vi "Master VI.vi"() -> ()   [LabVIEW 2010]
uses:
  <vilib>/Analysis/Matrix/Datatypes/RealMatrix.ctl
  Valve_Pump.ctl
  <vilib>/Analysis/Matrix/Comparison/Equal/Equal - RM,RM.vi
  <vilib>/Analysis/Matrix/NI_Matrix.lvlib
panel:
  in  "Density Profile":T1
  in  "Manual Override":bool
  in  "Drain Main Tank":bool
  in  "Open All":bool
  in  "Pump D":bool
  in  "V 37":bool
  in  "V 36":bool
  in  "V 35":bool
  in  "V 34":bool
  in  "V 32":bool
  in  "V 31":bool
  in  "V 28":bool
  in  "V 27":bool
  in  "V 26":bool
  in  "V 25":bool
  in  "V 24":bool
  in  "V 22":bool
  in  "V 21":bool
  in  "V 20":bool
  in  "V 18":bool
  in  "V 15":bool
  in  "V 14":bool
  in  "V 13":bool
  in  "V 12":bool
  in  "V 11":bool
  in  "V 10":bool
  in  "V 9":bool
  in  "V 8":bool
  in  "V 6":bool
  in  "V 5":bool
  in  "V 1":bool
  in  "Fill Main Tank":bool
  in  "V 23":bool
  in  "V 29":bool
  in  "V 30":bool
  in  "Pump A":bool
  out "Main tank":dbl(slide) scale=0.0..1.0
  out "Height of tank (m)":dbl
  out "Volume m^3*1000":i32
  in  "Reset":bool
  in  "Pump C":bool
  in  "Pump B":bool
  in  "V 19":bool
  in  "V 17":bool
  in  "V 16":bool
  in  "V 33":bool
  in  "V 3":bool
  in  "V 2":bool
  in  "V 4":bool
  in  "V 7":bool
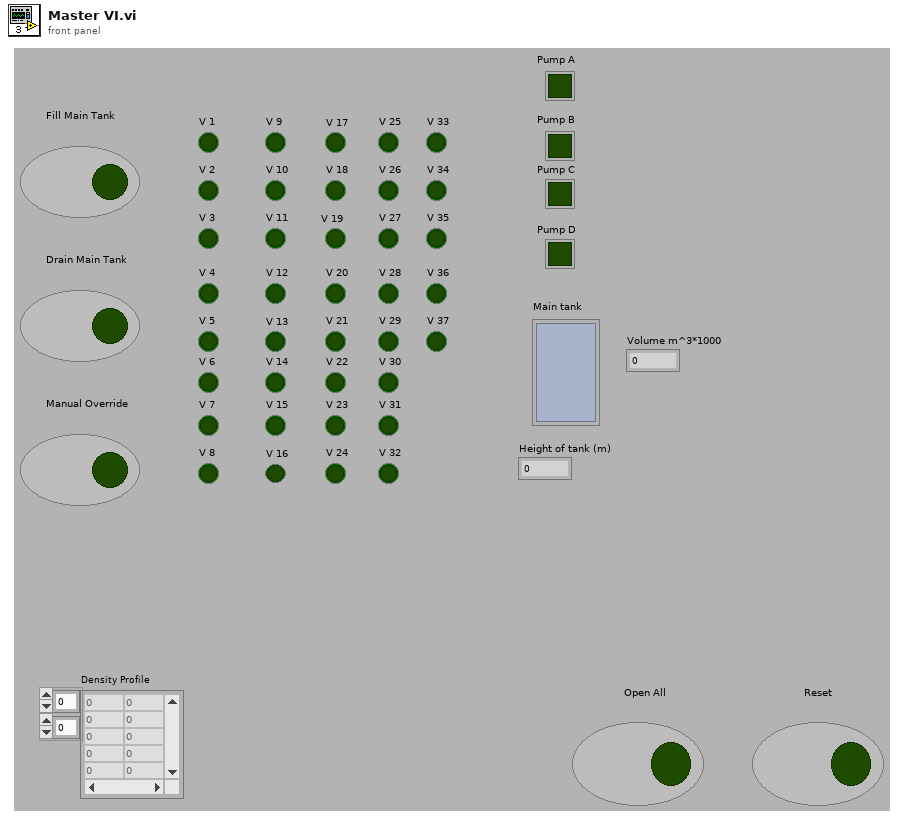
[diagram p1: front panel]
types:
  T1 = typedef "NI_Matrix.lvlib/RealMatrix.ctl" = dbl[][]
  T2 = typedef "Valve_Pump.ctl" = enum16{"V1", "V2", "V3", "V4", "V5", "V6", "V7", "V8", "V9", "V10", "V11", "V12", "V13", "V14", "V15", "V16", "V17", "V18", "V19", "V20", "V21", "V22", "V23", "V24", "V25", "V26", "V27", "V28", "V29", "V30", "V31", "V32", "V33", "V34", "V35", "V36", "V37", "Pump A", "Pump B", "Pump C", "Pump D"}
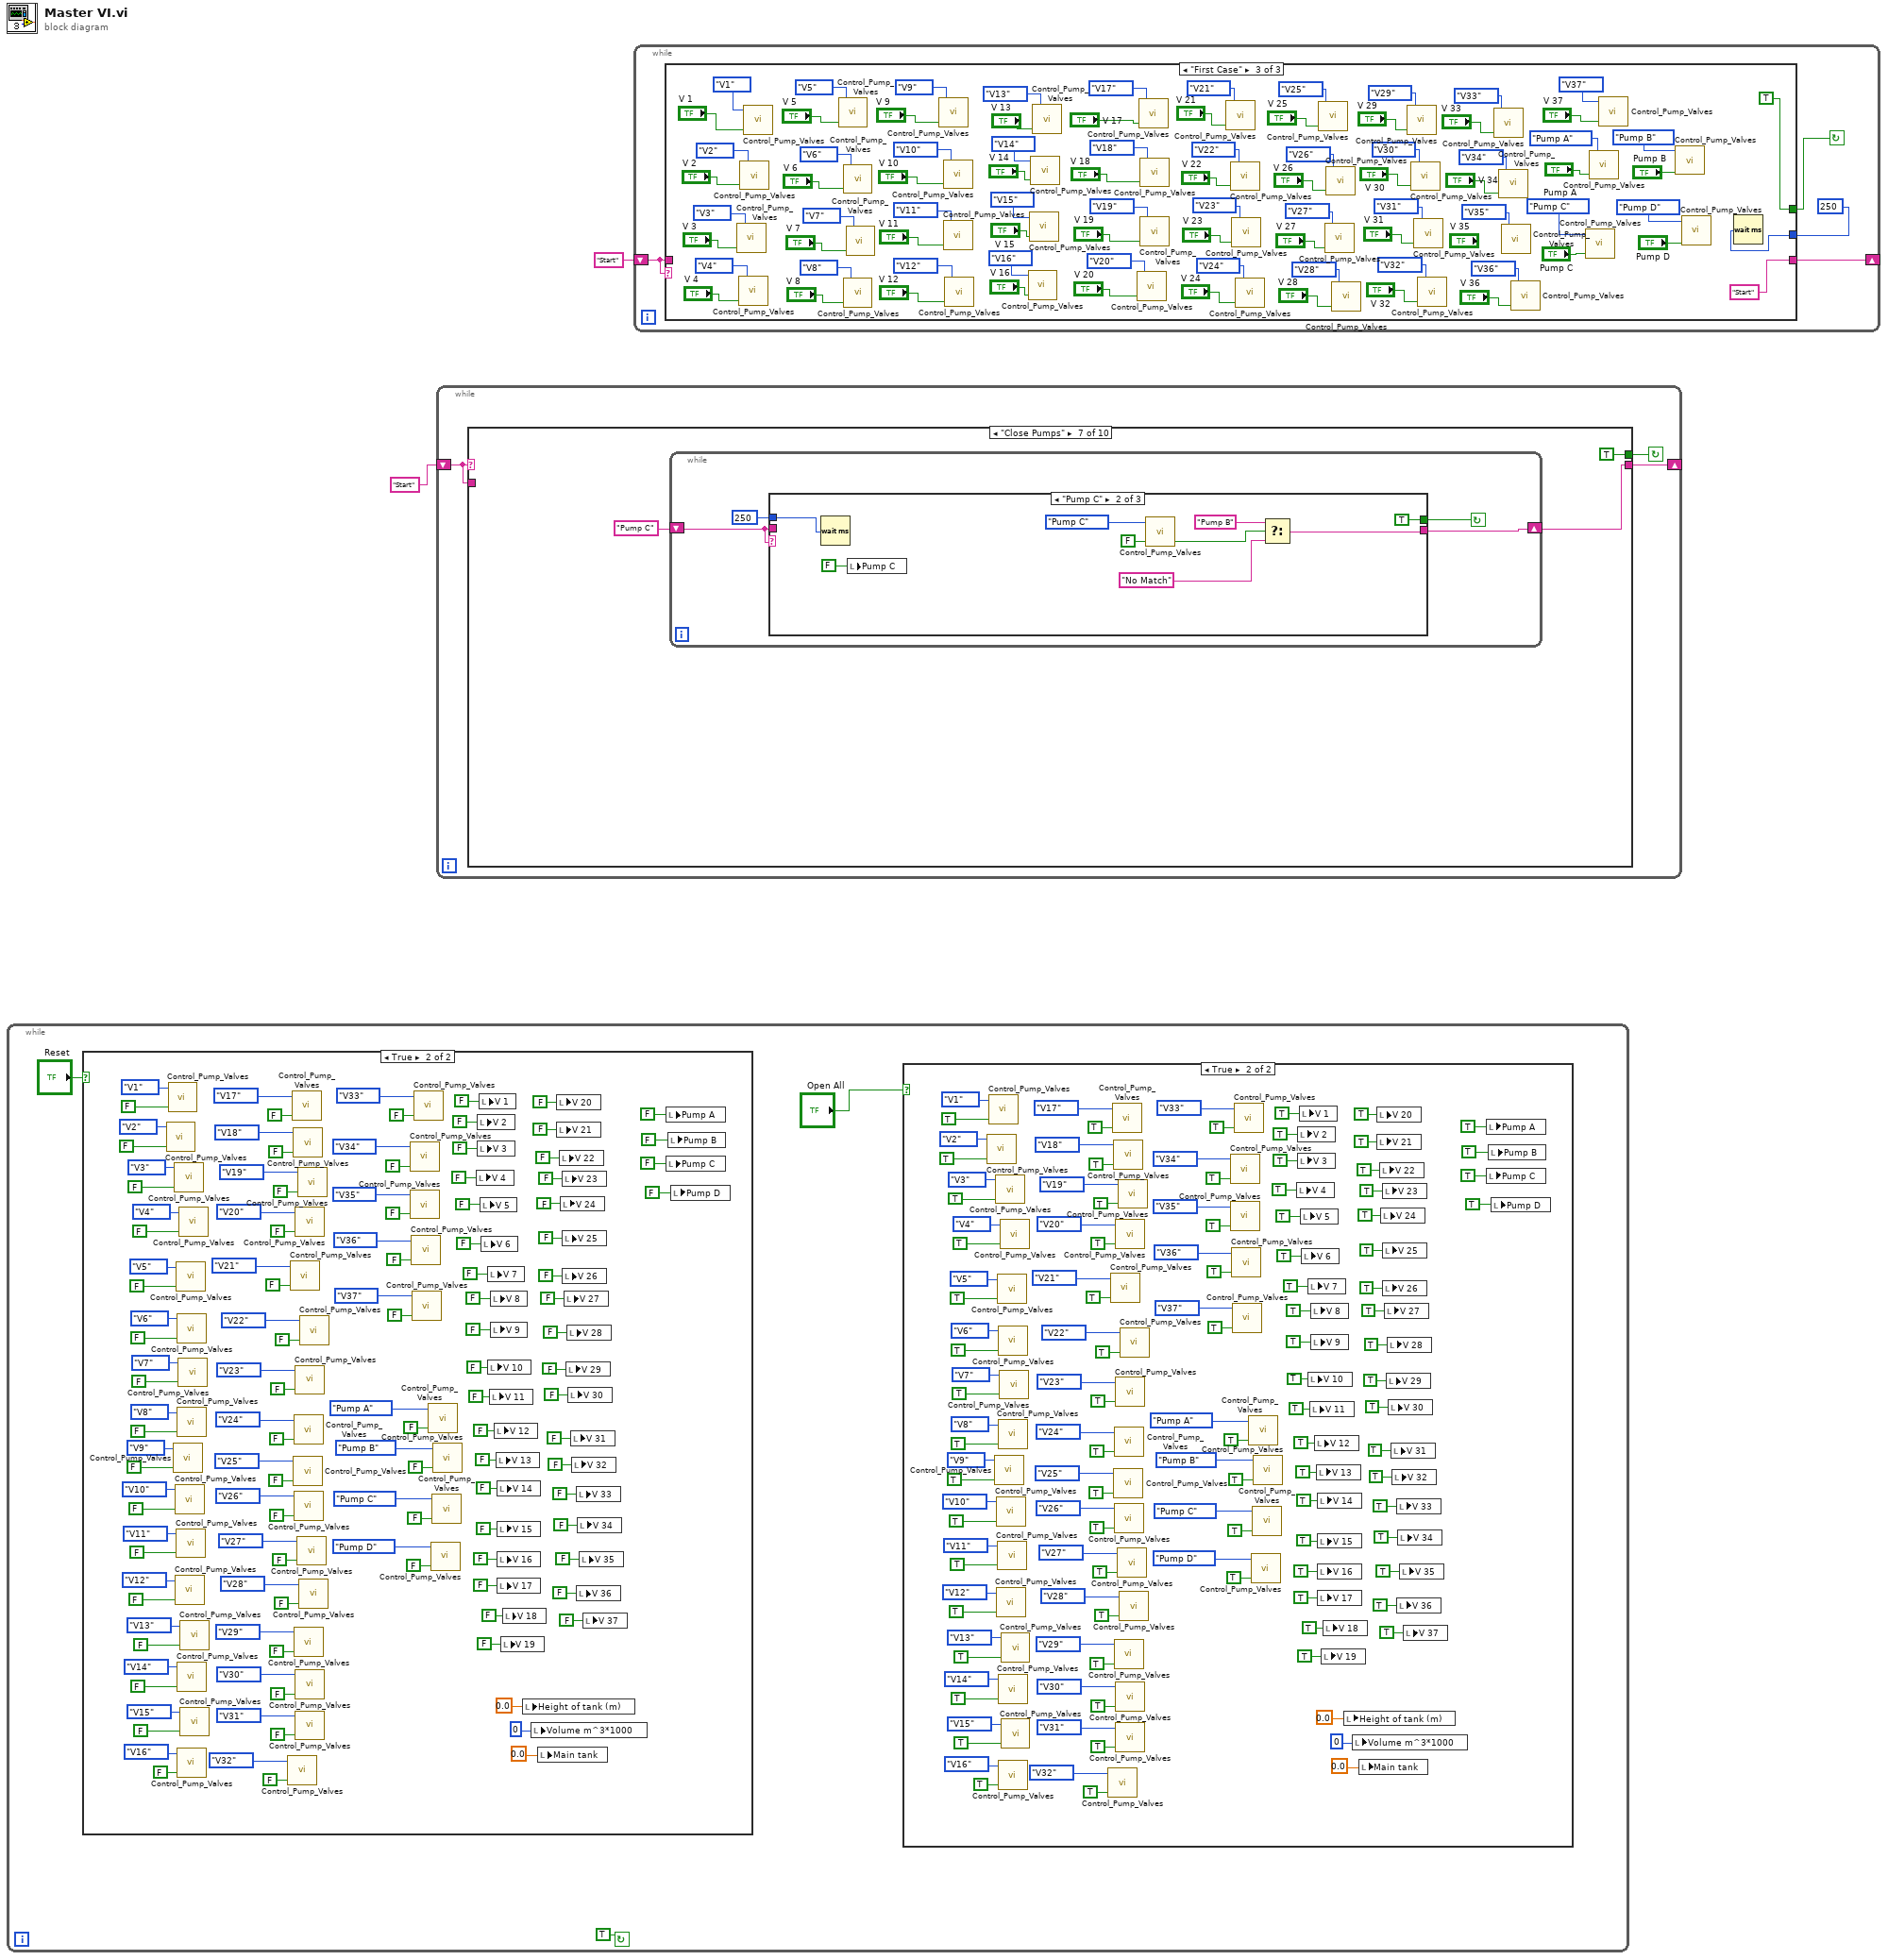
[diagram p0: block diagram]
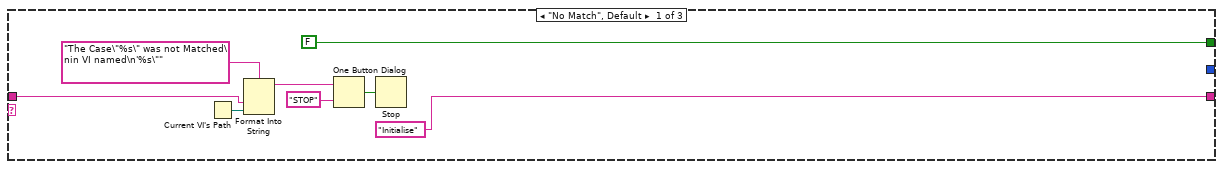
[diagram p2: hidden frame]
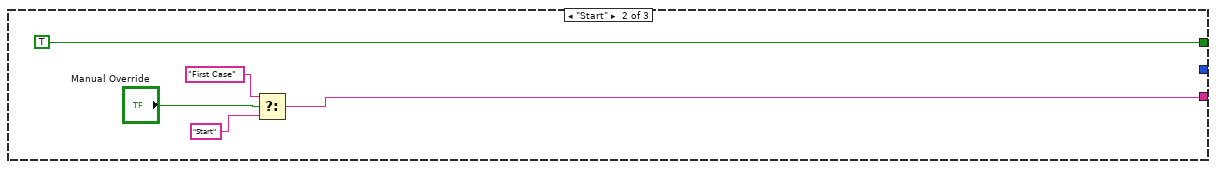
[diagram p3: hidden frame]
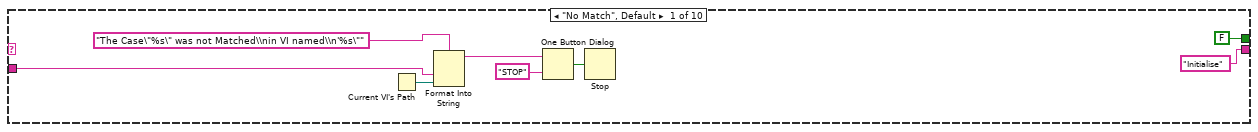
[diagram p6: hidden frame]
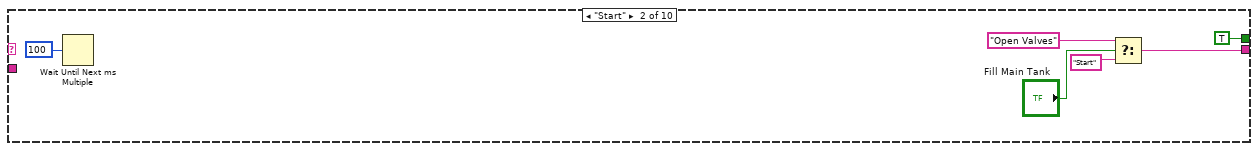
[diagram p7: hidden frame]
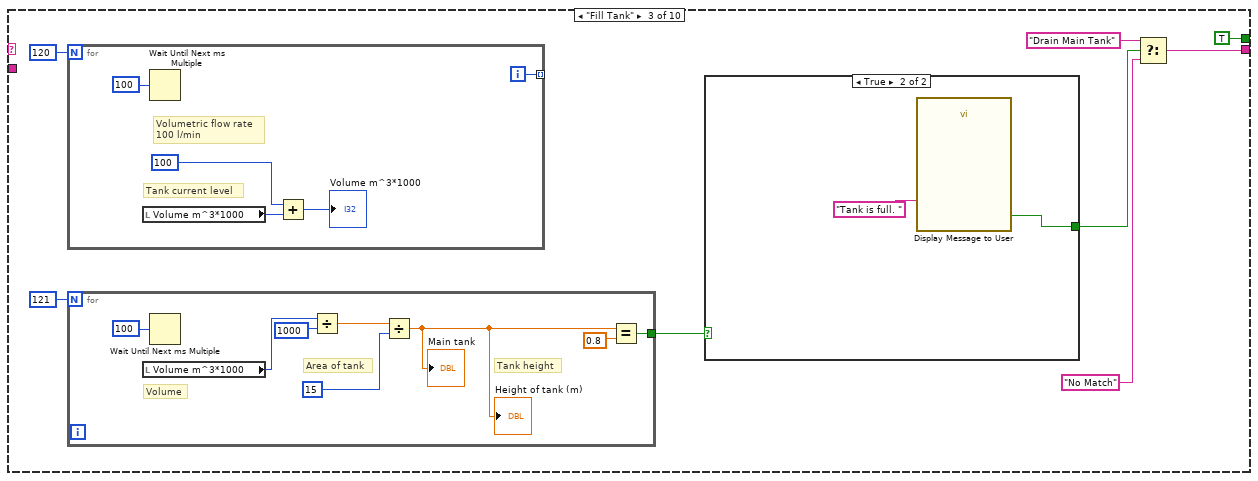
[diagram p8: hidden frame]
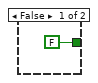
[diagram p9: hidden frame]
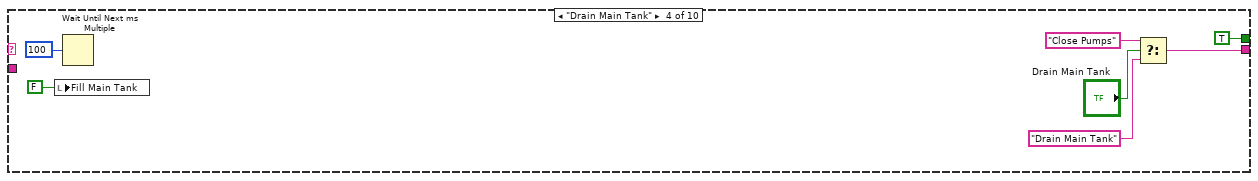
[diagram p10: hidden frame]
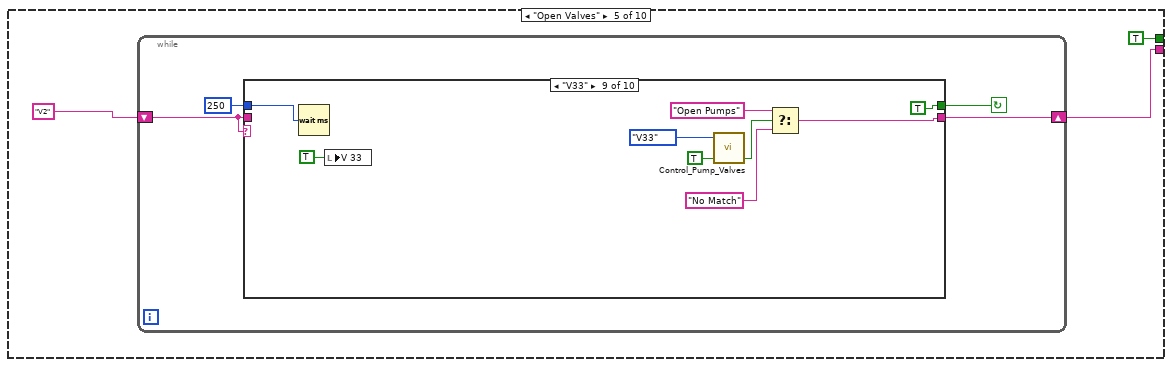
[diagram p11: hidden frame]
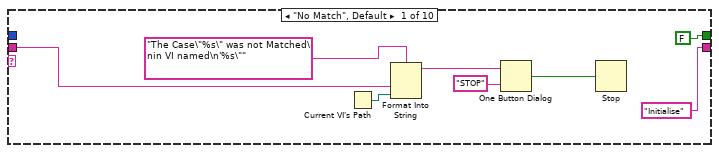
[diagram p12: hidden frame]
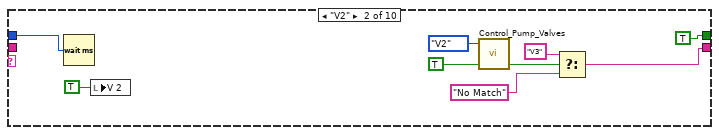
[diagram p13: hidden frame]
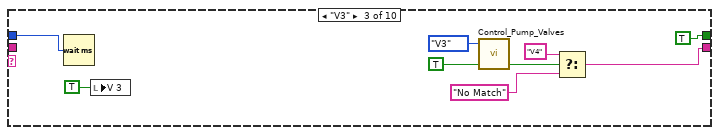
[diagram p14: hidden frame]
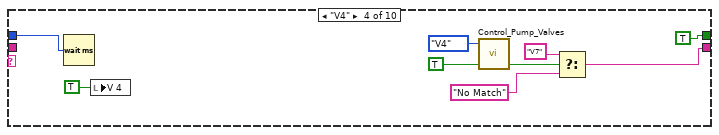
[diagram p15: hidden frame]
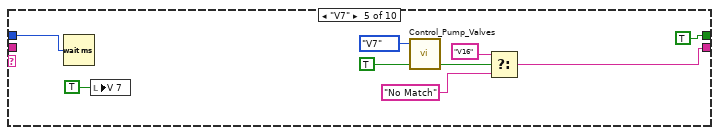
[diagram p16: hidden frame]
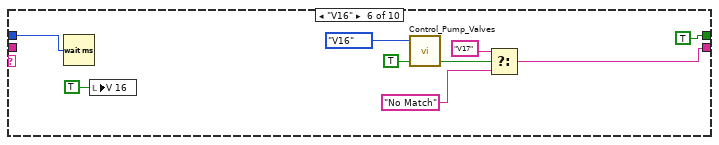
[diagram p17: hidden frame]
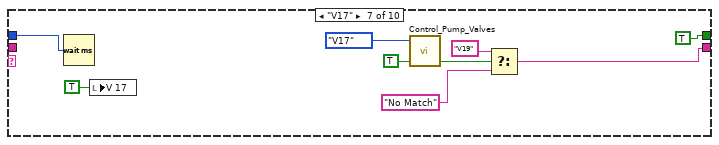
[diagram p18: hidden frame]
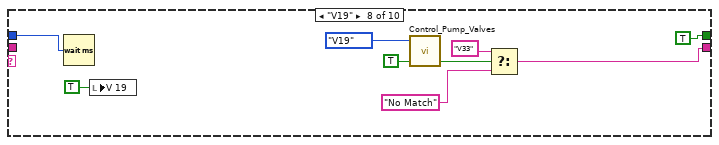
[diagram p19: hidden frame]
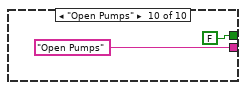
[diagram p20: hidden frame]
diagram:
  n1 = while {
    stop <- TRUE continue-if-true
    n2 = case shown="True" "Reset" {
      frame False {
      }
      frame True {
        n3 = call "Control_Pump_Valves.vi"("Set state:"=FALSE, "Device"=Valve_Pump."V2") -> ()  [unwired: 2 in, 2 out]
        n4 = call "Control_Pump_Valves.vi"("Set state:"=FALSE, "Device"=Valve_Pump."V1") -> ()  [unwired: 2 in, 2 out]
        n5 = call "Control_Pump_Valves.vi"("Set state:"=FALSE, "Device"=Valve_Pump."V9") -> ()  [unwired: 2 in, 2 out]
        n6 = call "Control_Pump_Valves.vi"("Set state:"=FALSE, "Device"=Valve_Pump."V3") -> ()  [unwired: 2 in, 2 out]
        n7 = call "Control_Pump_Valves.vi"("Set state:"=FALSE, "Device"=Valve_Pump."V10") -> ()  [unwired: 2 in, 2 out]
        n8 = call "Control_Pump_Valves.vi"("Set state:"=FALSE, "Device"=Valve_Pump."V12") -> ()  [unwired: 2 in, 2 out]
        n9 = call "Control_Pump_Valves.vi"("Set state:"=FALSE, "Device"=Valve_Pump."V5") -> ()  [unwired: 2 in, 2 out]
        n10 = call "Control_Pump_Valves.vi"("Set state:"=FALSE, "Device"=Valve_Pump."V11") -> ()  [unwired: 2 in, 2 out]
        n11 = call "Control_Pump_Valves.vi"("Set state:"=FALSE, "Device"=Valve_Pump."V6") -> ()  [unwired: 2 in, 2 out]
        n12 = call "Control_Pump_Valves.vi"("Set state:"=FALSE, "Device"=Valve_Pump."V8") -> ()  [unwired: 2 in, 2 out]
        n13 = call "Control_Pump_Valves.vi"("Set state:"=FALSE, "Device"=Valve_Pump."V14") -> ()  [unwired: 2 in, 2 out]
        n14 = call "Control_Pump_Valves.vi"("Set state:"=FALSE, "Device"=Valve_Pump."V16") -> ()  [unwired: 2 in, 2 out]
        n15 = call "Control_Pump_Valves.vi"("Set state:"=FALSE, "Device"=Valve_Pump."V7") -> ()  [unwired: 2 in, 2 out]
        n16 = call "Control_Pump_Valves.vi"("Set state:"=FALSE, "Device"=Valve_Pump."V4") -> ()  [unwired: 2 in, 2 out]
        n17 = call "Control_Pump_Valves.vi"("Set state:"=FALSE, "Device"=Valve_Pump."V13") -> ()  [unwired: 2 in, 2 out]
        n18 = call "Control_Pump_Valves.vi"("Set state:"=FALSE, "Device"=Valve_Pump."V15") -> ()  [unwired: 2 in, 2 out]
        n19 = call "Control_Pump_Valves.vi"("Set state:"=FALSE, "Device"=Valve_Pump."V32") -> ()  [unwired: 2 in, 2 out]
        n20 = call "Control_Pump_Valves.vi"("Set state:"=FALSE, "Device"=Valve_Pump."V21") -> ()  [unwired: 2 in, 2 out]
        n21 = call "Control_Pump_Valves.vi"("Set state:"=FALSE, "Device"=Valve_Pump."V17") -> ()  [unwired: 2 in, 2 out]
        n22 = call "Control_Pump_Valves.vi"("Set state:"=FALSE, "Device"=Valve_Pump."V18") -> ()  [unwired: 2 in, 2 out]
        n23 = call "Control_Pump_Valves.vi"("Set state:"=FALSE, "Device"=Valve_Pump."V25") -> ()  [unwired: 2 in, 2 out]
        n24 = call "Control_Pump_Valves.vi"("Set state:"=FALSE, "Device"=Valve_Pump."V24") -> ()  [unwired: 2 in, 2 out]
        n25 = call "Control_Pump_Valves.vi"("Set state:"=FALSE, "Device"=Valve_Pump."V26") -> ()  [unwired: 2 in, 2 out]
        n26 = call "Control_Pump_Valves.vi"("Set state:"=FALSE, "Device"=Valve_Pump."V29") -> ()  [unwired: 2 in, 2 out]
        n27 = call "Control_Pump_Valves.vi"("Set state:"=FALSE, "Device"=Valve_Pump."V20") -> ()  [unwired: 2 in, 2 out]
        n28 = call "Control_Pump_Valves.vi"("Set state:"=FALSE, "Device"=Valve_Pump."V23") -> ()  [unwired: 2 in, 2 out]
        n29 = call "Control_Pump_Valves.vi"("Set state:"=FALSE, "Device"=Valve_Pump."V30") -> ()  [unwired: 2 in, 2 out]
        n30 = call "Control_Pump_Valves.vi"("Set state:"=FALSE, "Device"=Valve_Pump."V31") -> ()  [unwired: 2 in, 2 out]
        n31 = call "Control_Pump_Valves.vi"("Set state:"=FALSE, "Device"=Valve_Pump."V27") -> ()  [unwired: 2 in, 2 out]
        n32 = call "Control_Pump_Valves.vi"("Set state:"=FALSE, "Device"=Valve_Pump."V19") -> ()  [unwired: 2 in, 2 out]
        n33 = call "Control_Pump_Valves.vi"("Set state:"=FALSE, "Device"=Valve_Pump."V28") -> ()  [unwired: 2 in, 2 out]
        n34 = call "Control_Pump_Valves.vi"("Set state:"=FALSE, "Device"=Valve_Pump."V22") -> ()  [unwired: 2 in, 2 out]
        n35 = call "Control_Pump_Valves.vi"("Set state:"=FALSE, "Device"=Valve_Pump."V34") -> ()  [unwired: 2 in, 2 out]
        n36 = call "Control_Pump_Valves.vi"("Set state:"=FALSE, "Device"=Valve_Pump."V35") -> ()  [unwired: 2 in, 2 out]
        n37 = call "Control_Pump_Valves.vi"("Set state:"=FALSE, "Device"=Valve_Pump."V36") -> ()  [unwired: 2 in, 2 out]
        n38 = call "Control_Pump_Valves.vi"("Set state:"=FALSE, "Device"=Valve_Pump."V37") -> ()  [unwired: 2 in, 2 out]
        n39 = call "Control_Pump_Valves.vi"("Set state:"=FALSE, "Device"=Valve_Pump."V33") -> ()  [unwired: 2 in, 2 out]
        n40 = call "Control_Pump_Valves.vi"("Set state:"=FALSE, "Device"=Valve_Pump."Pump A") -> ()  [unwired: 2 in, 2 out]
        n41 = call "Control_Pump_Valves.vi"("Set state:"=FALSE, "Device"=Valve_Pump."Pump D") -> ()  [unwired: 2 in, 2 out]
        n42 = call "Control_Pump_Valves.vi"("Set state:"=FALSE, "Device"=Valve_Pump."Pump C") -> ()  [unwired: 2 in, 2 out]
        n43 = call "Control_Pump_Valves.vi"("Set state:"=FALSE, "Device"=Valve_Pump."Pump B") -> ()  [unwired: 2 in, 2 out]
        n44 = local write "V 4"(FALSE ("V 4")) -> ()
        n45 = local write "V 2"(FALSE ("V 2")) -> ()
        n46 = local write "V 3"(FALSE ("V 3")) -> ()
        n47 = local write "V 1"(FALSE ("V 2")) -> ()
        n48 = local write "V 5"(FALSE ("V 3")) -> ()
        n49 = local write "V 6"(FALSE ("V 3")) -> ()
        n50 = local write "V 7"(FALSE ("V 7")) -> ()
        n51 = local write "V 10"(FALSE ("V 7")) -> ()
        n52 = local write "V 11"(FALSE ("V 7")) -> ()
        n53 = local write "V 8"(FALSE ("V 7")) -> ()
        n54 = local write "V 9"(FALSE ("V 7")) -> ()
        n55 = local write "V 12"(FALSE ("V 7")) -> ()
        n56 = local write "V 13"(FALSE ("V 7")) -> ()
        n57 = local write "V 14"(FALSE ("V 7")) -> ()
        n58 = local write "V 15"(FALSE ("V 7")) -> ()
        n59 = local write "V 16"(FALSE ("V 16")) -> ()
        n60 = local write "V 17"(FALSE ("V 17")) -> ()
        n61 = local write "V 19"(FALSE ("V 19")) -> ()
        n62 = local write "V 18"(FALSE ("V 7")) -> ()
        n63 = local write "Height of tank (m)"(0.0 ("Height of tank (m)")) -> ()
        n64 = local write "Volume m^3*1000"(0 ("Volume m^3*1000")) -> ()
        n65 = local write "Main tank"(0.0 ("Main tank")) -> ()
        n66 = local write "V 20"(FALSE ("V 19")) -> ()
        n67 = local write "V 21"(FALSE ("V 19")) -> ()
        n68 = local write "V 22"(FALSE ("V 19")) -> ()
        n69 = local write "V 24"(FALSE ("V 19")) -> ()
        n70 = local write "V 23"(FALSE ("V 19")) -> ()
        n71 = local write "V 25"(FALSE ("V 19")) -> ()
        n72 = local write "V 26"(FALSE ("V 19")) -> ()
        n73 = local write "V 27"(FALSE ("V 19")) -> ()
        n74 = local write "V 29"(FALSE ("V 19")) -> ()
        n75 = local write "V 28"(FALSE ("V 19")) -> ()
        n76 = local write "V 30"(FALSE ("V 19")) -> ()
        n77 = local write "V 31"(FALSE ("V 19")) -> ()
        n78 = local write "V 32"(FALSE ("V 33")) -> ()
        n79 = local write "V 33"(FALSE ("V 33")) -> ()
        n80 = local write "V 36"(FALSE ("V 19")) -> ()
        n81 = local write "V 34"(FALSE ("V 19")) -> ()
        n82 = local write "V 35"(FALSE ("V 19")) -> ()
        n83 = local write "V 37"(FALSE ("V 19")) -> ()
        n84 = local write "Pump A"(FALSE ("Pump B")) -> ()
        n85 = local write "Pump C"(FALSE ("Pump C")) -> ()
        n86 = local write "Pump B"(FALSE ("Pump B")) -> ()
        n87 = local write "Pump D"(FALSE ("Pump B")) -> ()
      }
    }
    n88 = case shown="True" "Open All" {
      frame False {
      }
      frame True {
        n89 = call "Control_Pump_Valves.vi"("Set state:"=TRUE, "Device"=Valve_Pump."V2") -> ()  [unwired: 2 in, 2 out]
        n90 = call "Control_Pump_Valves.vi"("Set state:"=TRUE, "Device"=Valve_Pump."V1") -> ()  [unwired: 2 in, 2 out]
        n91 = call "Control_Pump_Valves.vi"("Set state:"=TRUE, "Device"=Valve_Pump."V9") -> ()  [unwired: 2 in, 2 out]
        n92 = call "Control_Pump_Valves.vi"("Set state:"=TRUE, "Device"=Valve_Pump."V3") -> ()  [unwired: 2 in, 2 out]
        n93 = call "Control_Pump_Valves.vi"("Set state:"=TRUE, "Device"=Valve_Pump."V10") -> ()  [unwired: 2 in, 2 out]
        n94 = call "Control_Pump_Valves.vi"("Set state:"=TRUE, "Device"=Valve_Pump."V12") -> ()  [unwired: 2 in, 2 out]
        n95 = call "Control_Pump_Valves.vi"("Set state:"=TRUE, "Device"=Valve_Pump."V5") -> ()  [unwired: 2 in, 2 out]
        n96 = call "Control_Pump_Valves.vi"("Set state:"=TRUE, "Device"=Valve_Pump."V11") -> ()  [unwired: 2 in, 2 out]
        n97 = call "Control_Pump_Valves.vi"("Set state:"=TRUE, "Device"=Valve_Pump."V6") -> ()  [unwired: 2 in, 2 out]
        n98 = call "Control_Pump_Valves.vi"("Set state:"=TRUE, "Device"=Valve_Pump."V8") -> ()  [unwired: 2 in, 2 out]
        n99 = call "Control_Pump_Valves.vi"("Set state:"=TRUE, "Device"=Valve_Pump."V14") -> ()  [unwired: 2 in, 2 out]
        n100 = call "Control_Pump_Valves.vi"("Set state:"=TRUE, "Device"=Valve_Pump."V16") -> ()  [unwired: 2 in, 2 out]
        n101 = call "Control_Pump_Valves.vi"("Set state:"=TRUE, "Device"=Valve_Pump."V7") -> ()  [unwired: 2 in, 2 out]
        n102 = call "Control_Pump_Valves.vi"("Set state:"=TRUE, "Device"=Valve_Pump."V4") -> ()  [unwired: 2 in, 2 out]
        n103 = call "Control_Pump_Valves.vi"("Set state:"=TRUE, "Device"=Valve_Pump."V13") -> ()  [unwired: 2 in, 2 out]
        n104 = call "Control_Pump_Valves.vi"("Set state:"=TRUE, "Device"=Valve_Pump."V15") -> ()  [unwired: 2 in, 2 out]
        n105 = call "Control_Pump_Valves.vi"("Set state:"=TRUE, "Device"=Valve_Pump."V32") -> ()  [unwired: 2 in, 2 out]
        n106 = call "Control_Pump_Valves.vi"("Set state:"=TRUE, "Device"=Valve_Pump."V21") -> ()  [unwired: 2 in, 2 out]
        n107 = call "Control_Pump_Valves.vi"("Set state:"=TRUE, "Device"=Valve_Pump."V17") -> ()  [unwired: 2 in, 2 out]
        n108 = call "Control_Pump_Valves.vi"("Set state:"=TRUE, "Device"=Valve_Pump."V18") -> ()  [unwired: 2 in, 2 out]
        n109 = call "Control_Pump_Valves.vi"("Set state:"=TRUE, "Device"=Valve_Pump."V25") -> ()  [unwired: 2 in, 2 out]
        n110 = call "Control_Pump_Valves.vi"("Set state:"=TRUE, "Device"=Valve_Pump."V24") -> ()  [unwired: 2 in, 2 out]
        n111 = call "Control_Pump_Valves.vi"("Set state:"=TRUE, "Device"=Valve_Pump."V26") -> ()  [unwired: 2 in, 2 out]
        n112 = call "Control_Pump_Valves.vi"("Set state:"=TRUE, "Device"=Valve_Pump."V29") -> ()  [unwired: 2 in, 2 out]
        n113 = call "Control_Pump_Valves.vi"("Set state:"=TRUE, "Device"=Valve_Pump."V20") -> ()  [unwired: 2 in, 2 out]
        n114 = call "Control_Pump_Valves.vi"("Set state:"=TRUE, "Device"=Valve_Pump."V23") -> ()  [unwired: 2 in, 2 out]
        n115 = call "Control_Pump_Valves.vi"("Set state:"=TRUE, "Device"=Valve_Pump."V30") -> ()  [unwired: 2 in, 2 out]
        n116 = call "Control_Pump_Valves.vi"("Set state:"=TRUE, "Device"=Valve_Pump."V31") -> ()  [unwired: 2 in, 2 out]
        n117 = call "Control_Pump_Valves.vi"("Set state:"=TRUE, "Device"=Valve_Pump."V27") -> ()  [unwired: 2 in, 2 out]
        n118 = call "Control_Pump_Valves.vi"("Set state:"=TRUE, "Device"=Valve_Pump."V19") -> ()  [unwired: 2 in, 2 out]
        n119 = call "Control_Pump_Valves.vi"("Set state:"=TRUE, "Device"=Valve_Pump."V28") -> ()  [unwired: 2 in, 2 out]
        n120 = call "Control_Pump_Valves.vi"("Set state:"=TRUE, "Device"=Valve_Pump."V22") -> ()  [unwired: 2 in, 2 out]
        n121 = call "Control_Pump_Valves.vi"("Set state:"=TRUE, "Device"=Valve_Pump."V34") -> ()  [unwired: 2 in, 2 out]
        n122 = call "Control_Pump_Valves.vi"("Set state:"=TRUE, "Device"=Valve_Pump."V35") -> ()  [unwired: 2 in, 2 out]
        n123 = call "Control_Pump_Valves.vi"("Set state:"=TRUE, "Device"=Valve_Pump."V36") -> ()  [unwired: 2 in, 2 out]
        n124 = call "Control_Pump_Valves.vi"("Set state:"=TRUE, "Device"=Valve_Pump."V37") -> ()  [unwired: 2 in, 2 out]
        n125 = call "Control_Pump_Valves.vi"("Set state:"=TRUE, "Device"=Valve_Pump."V33") -> ()  [unwired: 2 in, 2 out]
        n126 = call "Control_Pump_Valves.vi"("Set state:"=TRUE, "Device"=Valve_Pump."Pump A") -> ()  [unwired: 2 in, 2 out]
        n127 = call "Control_Pump_Valves.vi"("Set state:"=TRUE, "Device"=Valve_Pump."Pump D") -> ()  [unwired: 2 in, 2 out]
        n128 = call "Control_Pump_Valves.vi"("Set state:"=TRUE, "Device"=Valve_Pump."Pump C") -> ()  [unwired: 2 in, 2 out]
        n129 = call "Control_Pump_Valves.vi"("Set state:"=TRUE, "Device"=Valve_Pump."Pump B") -> ()  [unwired: 2 in, 2 out]
        n130 = local write "V 4"(TRUE ("V 4")) -> ()
        n131 = local write "V 2"(TRUE ("V 2")) -> ()
        n132 = local write "V 3"(TRUE ("V 3")) -> ()
        n133 = local write "V 1"(TRUE ("V 2")) -> ()
        n134 = local write "V 5"(TRUE ("V 3")) -> ()
        n135 = local write "V 6"(TRUE ("V 3")) -> ()
        n136 = local write "V 7"(TRUE ("V 7")) -> ()
        n137 = local write "V 10"(TRUE ("V 7")) -> ()
        n138 = local write "V 11"(TRUE ("V 7")) -> ()
        n139 = local write "V 8"(TRUE ("V 7")) -> ()
        n140 = local write "V 9"(TRUE ("V 7")) -> ()
        n141 = local write "V 12"(TRUE ("V 7")) -> ()
        n142 = local write "V 13"(TRUE ("V 7")) -> ()
        n143 = local write "V 14"(TRUE ("V 7")) -> ()
        n144 = local write "V 15"(TRUE ("V 7")) -> ()
        n145 = local write "V 16"(TRUE ("V 16")) -> ()
        n146 = local write "V 17"(TRUE ("V 17")) -> ()
        n147 = local write "V 19"(TRUE ("V 19")) -> ()
        n148 = local write "V 18"(TRUE ("V 7")) -> ()
        n149 = local write "Height of tank (m)"(0.0 ("Height of tank (m)")) -> ()
        n150 = local write "Volume m^3*1000"(0 ("Volume m^3*1000")) -> ()
        n151 = local write "Main tank"(0.0 ("Main tank")) -> ()
        n152 = local write "V 20"(TRUE ("V 19")) -> ()
        n153 = local write "V 21"(TRUE ("V 19")) -> ()
        n154 = local write "V 22"(TRUE ("V 19")) -> ()
        n155 = local write "V 24"(TRUE ("V 19")) -> ()
        n156 = local write "V 23"(TRUE ("V 19")) -> ()
        n157 = local write "V 25"(TRUE ("V 19")) -> ()
        n158 = local write "V 26"(TRUE ("V 19")) -> ()
        n159 = local write "V 27"(TRUE ("V 19")) -> ()
        n160 = local write "V 29"(TRUE ("V 19")) -> ()
        n161 = local write "V 28"(TRUE ("V 19")) -> ()
        n162 = local write "V 30"(TRUE ("V 19")) -> ()
        n163 = local write "V 31"(TRUE ("V 19")) -> ()
        n164 = local write "V 32"(TRUE ("V 33")) -> ()
        n165 = local write "V 33"(TRUE ("V 33")) -> ()
        n166 = local write "V 36"(TRUE ("V 19")) -> ()
        n167 = local write "V 34"(TRUE ("V 19")) -> ()
        n168 = local write "V 35"(TRUE ("V 19")) -> ()
        n169 = local write "V 37"(TRUE ("V 19")) -> ()
        n170 = local write "Pump A"(TRUE ("Pump B")) -> ()
        n171 = local write "Pump C"(TRUE ("Pump C")) -> ()
        n172 = local write "Pump B"(TRUE ("Pump B")) -> ()
        n173 = local write "Pump D"(TRUE ("Pump B")) -> ()
      }
    }
  }
  n174 = while {
    shift-left: "Start" -> [w258]
    shift-right: [w259] -> _
    stop <- w260 continue-if-true
    n175 = case shown="\"Close Pumps\"" w258 {
      tunnel: [FALSE TRUE TRUE TRUE TRUE TRUE TRUE TRUE TRUE TRUE] -> w260
      tunnel: ["Initialise" w271 w275 w301 w306 w395 w436 w469 w583 w607] -> w259
      tunnel: w258 -> [w263 _ _ _ _ _ _ _ _ _]
      frame "No Match", Default {
        n176 = Current VI's Path() -> (path=w262:path)
        n177 = Format Into String(format string="The Case\"%s\" was not Matched\\nin VI named\\n'%s\"" ("Format String"), w263, w262) -> (resulting string=w266:string)  [unwired: 2 in, 1 out]
        n178 = One Button Dialog(message=w266, button name ("OK")="STOP") -> (true=w264:bool)
        n179 = Stop(stop? (T)=w264) -> ()
      }
      frame "Start" {
        n180 = Wait Until Next ms Multiple(millisecond multiple=u32 100) -> ()  [unwired: 1 out]
        n181 = Select(t="Open Valves", s="Fill Main Tank", f="Start") -> (s? t:f=w271:string)
      }
      frame "Fill Tank" {
        n182 = for {
          N: 120 -> [_]
          tunnel: [w294] -> _ mode=indexing
          i -> [w294]
          # "Tank current level"
          # "Volumetric flow rate\n100 l/min"
          n183 = local read "Volume m^3*1000"() -> (w297:i32)
          n184 = Wait Until Next ms Multiple(millisecond multiple=u32 100) -> ()  [unwired: 1 out]
          n185 = Add(x=100, y=w297) -> (x+y=→"Volume m^3*1000":i32)
        }
        n186 = for {
          N: 121 -> [_]
          tunnel: [w283] -> w281
          # "Volume"
          # "Tank height"
          # "Area of tank"
          n187 = local read "Volume m^3*1000"() -> (w289:i32)
          n188 = Wait Until Next ms Multiple(millisecond multiple=u32 100 ("milliseconds to wait")) -> ()  [unwired: 1 out]
          n189 = Divide(x=w289, y=1000) -> (x/y=w287:dbl)
          n190 = Divide(x=w287, y=15) -> (x/y=w284:dbl)
          "Main tank" <- w284
          "Height of tank (m)" <- w284
          n191 = Equal?(x=w284, y=0.8) -> (x = y?=w283:bool)
        }
        n192 = case shown="True" w281 {
          tunnel: [FALSE ("OK") w292] -> w278
          frame False {
          }
          frame True {
            n193 = call "Display Message to User"("Message"="Tank is full. ") -> ("OK"=w292:bool)  [unwired: 9 in, 1 out]
          }
        }
        n194 = Select(t="Drain Main Tank" ("Message"), s=w278, f="No Match" ("Message")) -> (s? t:f=w275:string)
      }
      frame "Drain Main Tank" {
        n195 = local write "Fill Main Tank"(FALSE ("Fill Main Tank")) -> ()
        n196 = Wait Until Next ms Multiple(millisecond multiple=u32 100) -> ()  [unwired: 1 out]
        n197 = Select(t="Close Pumps", s="Drain Main Tank", f="Drain Main Tank") -> (s? t:f=w301:string)
      }
      frame "Open Valves" {
        n198 = while {
          shift-left: "V2" -> [w310]
          shift-right: [w311] -> w306
          stop <- w312 continue-if-true
          n199 = case shown="\"V33\"" w310 {
            tunnel: [FALSE TRUE TRUE TRUE TRUE TRUE TRUE TRUE TRUE FALSE] -> w312
            tunnel: ["Initialise" w323 w332 w341 w350 w359 w368 w377 w386 "Open Pumps" ("Message")] -> w311
            tunnel: w310 -> [w315 _ _ _ _ _ _ _ _ _]
            tunnel: u32 250 ("milliseconds to wait") -> [_ w327 w335 w344 w353 w362 w371 w380 w389 _]
            frame "No Match", Default {
              n200 = Current VI's Path() -> (path=w314:path)
              n201 = Format Into String(format string="The Case\"%s\" was not Matched\nin VI named\n'%s\"" ("Format String"), w315, w314) -> (resulting string=w318:string)  [unwired: 2 in, 1 out]
              n202 = One Button Dialog(message=w318, button name ("OK")="STOP") -> (true=w316:bool)
              n203 = Stop(stop? (T)=w316) -> ()
            }
            frame "V2" {
              n204 = Wait (ms)(milliseconds to wait=w327) -> ()  [unwired: 1 out]
              n205 = local write "V 2"(TRUE ("V 2")) -> ()
              n206 = call "Control_Pump_Valves.vi"("Set state:"=TRUE, "Device"=Valve_Pump."V2") -> ("Good Reply"=w322:bool)  [unwired: 2 in, 1 out]
              n207 = Select(t="V3", s=w322, f="No Match" ("Message")) -> (s? t:f=w323:string)
            }
            frame "V3" {
              n208 = Wait (ms)(milliseconds to wait=w335) -> ()  [unwired: 1 out]
              n209 = local write "V 3"(TRUE ("V 3")) -> ()
              n210 = call "Control_Pump_Valves.vi"("Set state:"=TRUE, "Device"=Valve_Pump."V3") -> ("Good Reply"=w331:bool)  [unwired: 2 in, 1 out]
              n211 = Select(t="V4", s=w331, f="No Match" ("Message")) -> (s? t:f=w332:string)
            }
            frame "V4" {
              n212 = Wait (ms)(milliseconds to wait=w344) -> ()  [unwired: 1 out]
              n213 = local write "V 4"(TRUE ("V 4")) -> ()
              n214 = call "Control_Pump_Valves.vi"("Set state:"=TRUE, "Device"=Valve_Pump."V4") -> ("Good Reply"=w340:bool)  [unwired: 2 in, 1 out]
              n215 = Select(t="V7", s=w340, f="No Match" ("Message")) -> (s? t:f=w341:string)
            }
            frame "V7" {
              n216 = Wait (ms)(milliseconds to wait=w353) -> ()  [unwired: 1 out]
              n217 = local write "V 7"(TRUE ("V 7")) -> ()
              n218 = call "Control_Pump_Valves.vi"("Set state:"=TRUE, "Device"=Valve_Pump."V7") -> ("Good Reply"=w349:bool)  [unwired: 2 in, 1 out]
              n219 = Select(t="V16", s=w349, f="No Match" ("Message")) -> (s? t:f=w350:string)
            }
            frame "V16" {
              n220 = Wait (ms)(milliseconds to wait=w362) -> ()  [unwired: 1 out]
              n221 = local write "V 16"(TRUE ("V 3")) -> ()
              n222 = call "Control_Pump_Valves.vi"("Set state:"=TRUE, "Device"=Valve_Pump."V16") -> ("Good Reply"=w358:bool)  [unwired: 2 in, 1 out]
              n223 = Select(t="V17", s=w358, f="No Match" ("Message")) -> (s? t:f=w359:string)
            }
            frame "V17" {
              n224 = Wait (ms)(milliseconds to wait=w371) -> ()  [unwired: 1 out]
              n225 = local write "V 17"(TRUE ("V 3")) -> ()
              n226 = call "Control_Pump_Valves.vi"("Set state:"=TRUE, "Device"=Valve_Pump."V17") -> ("Good Reply"=w367:bool)  [unwired: 2 in, 1 out]
              n227 = Select(t="V19", s=w367, f="No Match" ("Message")) -> (s? t:f=w368:string)
            }
            frame "V19" {
              n228 = Wait (ms)(milliseconds to wait=w380) -> ()  [unwired: 1 out]
              n229 = local write "V 19"(TRUE ("V 3")) -> ()
              n230 = call "Control_Pump_Valves.vi"("Set state:"=TRUE, "Device"=Valve_Pump."V19") -> ("Good Reply"=w376:bool)  [unwired: 2 in, 1 out]
              n231 = Select(t="V33", s=w376, f="No Match" ("Message")) -> (s? t:f=w377:string)
            }
            frame "V33" {
              n232 = Wait (ms)(milliseconds to wait=w389) -> ()  [unwired: 1 out]
              n233 = local write "V 33"(TRUE ("V 3")) -> ()
              n234 = call "Control_Pump_Valves.vi"("Set state:"=TRUE, "Device"=Valve_Pump."V33") -> ("Good Reply"=w385:bool)  [unwired: 2 in, 1 out]
              n235 = Select(t="Open Pumps", s=w385, f="No Match" ("Message")) -> (s? t:f=w386:string)
            }
            frame "Open Pumps" {
            }
          }
        }
      }
      frame "Open Pumps" {
        n236 = while {
          shift-left: "Pump B" -> [w399]
          shift-right: [w400] -> w395
          stop <- w401 continue-if-true
          n237 = case shown="\"Pump C\"" w399 {
            tunnel: [FALSE TRUE TRUE FALSE] -> w401
            tunnel: ["Initialise" w412 w421 w431] -> w400
            tunnel: w399 -> [w404 _ _ _]
            tunnel: u32 250 ("milliseconds to wait") -> [_ w416 w424 w434]
            frame "No Match", Default {
              n238 = Current VI's Path() -> (path=w403:path)
              n239 = Format Into String(format string="The Case\"%s\" was not Matched\nin VI named\n'%s\"" ("Format String"), w404, w403) -> (resulting string=w407:string)  [unwired: 2 in, 1 out]
              n240 = One Button Dialog(message=w407, button name ("OK")="STOP") -> (true=w405:bool)
              n241 = Stop(stop? (T)=w405) -> ()
            }
            frame "Pump B" {
              n242 = Wait (ms)(milliseconds to wait=w416) -> ()  [unwired: 1 out]
              n243 = local write "Pump B"(TRUE ("Pump B")) -> ()
              n244 = call "Control_Pump_Valves.vi"("Set state:"=TRUE, "Device"=Valve_Pump."Pump B") -> ("Good Reply"=w411:bool)  [unwired: 2 in, 1 out]
              n245 = Select(t="Pump C", s=w411, f="No Match" ("Message")) -> (s? t:f=w412:string)
            }
            frame "Pump C" {
              n246 = Wait (ms)(milliseconds to wait=w424) -> ()  [unwired: 1 out]
              n247 = local write "Pump C"(TRUE ("Pump B")) -> ()
              n248 = call "Control_Pump_Valves.vi"("Set state:"=TRUE, "Device"=Valve_Pump."Pump C") -> ("Good Reply"=w420:bool)  [unwired: 2 in, 1 out]
              n249 = Select(t="Density Profile", s=w420, f="No Match" ("Message")) -> (s? t:f=w421:string)
            }
            frame "Density Profile" {
              n250 = Wait (ms)(milliseconds to wait=w434) -> ()  [unwired: 1 out]
              n251 = call-poly <vilib>:"Equal.vi"("Real Matrix B"=T1 [[1200.0, 0.0], [1150.0, 0.2], [1100.0, 0.4], [1050.0, 0.6], [1000.0, 0.8]] ("Density Profile 2"), "Real Matrix A"="Density Profile") -> ("A = B?"=w428:bool)
              n252 = Select(t="Fill Tank", s=w428, f="No Match" ("Message")) -> (s? t:f=w431:string)
            }
          }
        }
      }
      frame "Close Pumps" {
        n253 = while {
          shift-left: "Pump C" -> [w440]
          shift-right: [w441] -> w436
          stop <- w442 continue-if-true
          n254 = case shown="\"Pump C\"" w440 {
            tunnel: [FALSE TRUE FALSE] -> w442
            tunnel: ["Initialise" w453 w462] -> w441
            tunnel: w440 -> [w445 _ _]
            tunnel: u32 250 ("milliseconds to wait") -> [_ w456 w466]
            frame "No Match", Default {
              n255 = Current VI's Path() -> (path=w444:path)
              n256 = Format Into String(format string="The Case\"%s\" was not Matched\nin VI named\n'%s\"" ("Format String"), w445, w444) -> (resulting string=w448:string)  [unwired: 2 in, 1 out]
              n257 = One Button Dialog(message=w448, button name ("OK")="STOP") -> (true=w446:bool)
              n258 = Stop(stop? (T)=w446) -> ()
            }
            frame "Pump C" {
              n259 = Wait (ms)(milliseconds to wait=w456) -> ()  [unwired: 1 out]
              n260 = local write "Pump C"(FALSE ("Pump B")) -> ()
              n261 = call "Control_Pump_Valves.vi"("Set state:"=FALSE, "Device"=Valve_Pump."Pump C") -> ("Good Reply"=w452:bool)  [unwired: 2 in, 1 out]
              n262 = Select(t="Pump B", s=w452, f="No Match" ("Message")) -> (s? t:f=w453:string)
            }
            frame "Pump B" {
              n263 = Wait (ms)(milliseconds to wait=w466) -> ()  [unwired: 1 out]
              n264 = local write "Pump B"(FALSE ("Pump B")) -> ()
              n265 = call "Control_Pump_Valves.vi"("Set state:"=FALSE, "Device"=Valve_Pump."Pump B") -> ("Good Reply"=w461:bool)  [unwired: 2 in, 1 out]
              n266 = Select(t="Close Valves", s=w461, f="No Match" ("Message")) -> (s? t:f=w462:string)
            }
          }
        }
      }
      frame "Close Valves" {
        n267 = while {
          shift-left: "V2" -> [w473]
          shift-right: [w474] -> w469
          stop <- w475 continue-if-true
          n268 = case shown="\"Pump A\"" w473 {
            tunnel: [FALSE TRUE TRUE TRUE TRUE TRUE TRUE TRUE TRUE TRUE TRUE FALSE] -> w475
            tunnel: ["Initialise" w486 w495 w504 w513 w522 w531 w540 w549 w558 w567 w576] -> w474
            tunnel: w473 -> [w478 _ _ _ _ _ _ _ _ _ _ _]
            tunnel: u32 250 ("milliseconds to wait") -> [_ w489 w499 w508 w517 w526 w535 w544 w553 w562 w571 w580]
            frame "No Match", Default {
              n269 = Current VI's Path() -> (path=w477:path)
              n270 = Format Into String(format string="The Case\"%s\" was not Matched\nin VI named\n'%s\"" ("Format String"), w478, w477) -> (resulting string=w481:string)  [unwired: 2 in, 1 out]
              n271 = One Button Dialog(message=w481, button name ("OK")="STOP") -> (true=w479:bool)
              n272 = Stop(stop? (T)=w479) -> ()
            }
            frame "V2" {
              n273 = Wait (ms)(milliseconds to wait=w489) -> ()  [unwired: 1 out]
              n274 = local write "V 2"(FALSE ("V 4")) -> ()
              n275 = call "Control_Pump_Valves.vi"("Set state:"=FALSE, "Device"=Valve_Pump."V2") -> ("Good Reply"=w485:bool)  [unwired: 2 in, 1 out]
              n276 = Select(t="V3", s=w485, f="No Match" ("Message")) -> (s? t:f=w486:string)
            }
            frame "V3" {
              n277 = Wait (ms)(milliseconds to wait=w499) -> ()  [unwired: 1 out]
              n278 = local write "V 3"(FALSE ("V 3")) -> ()
              n279 = call "Control_Pump_Valves.vi"("Set state:"=FALSE, "Device"=Valve_Pump."V3") -> ("Good Reply"=w494:bool)  [unwired: 2 in, 1 out]
              n280 = Select(t="V4", s=w494, f="No Match" ("Message")) -> (s? t:f=w495:string)
            }
            frame "V4" {
              n281 = Wait (ms)(milliseconds to wait=w508) -> ()  [unwired: 1 out]
              n282 = local write "V 4"(FALSE ("V 3")) -> ()
              n283 = call "Control_Pump_Valves.vi"("Set state:"=FALSE, "Device"=Valve_Pump."V4") -> ("Good Reply"=w503:bool)  [unwired: 2 in, 1 out]
              n284 = Select(t="V7", s=w503, f="No Match" ("Message")) -> (s? t:f=w504:string)
            }
            frame "V7" {
              n285 = Wait (ms)(milliseconds to wait=w517) -> ()  [unwired: 1 out]
              n286 = local write "V 7"(FALSE ("V 3")) -> ()
              n287 = call "Control_Pump_Valves.vi"("Set state:"=FALSE, "Device"=Valve_Pump."V7") -> ("Good Reply"=w512:bool)  [unwired: 2 in, 1 out]
              n288 = Select(t="V16", s=w512, f="No Match" ("Message")) -> (s? t:f=w513:string)
            }
            frame "V16" {
              n289 = Wait (ms)(milliseconds to wait=w526) -> ()  [unwired: 1 out]
              n290 = local write "V 16"(FALSE ("V 3")) -> ()
              n291 = call "Control_Pump_Valves.vi"("Set state:"=FALSE, "Device"=Valve_Pump."V16") -> ("Good Reply"=w521:bool)  [unwired: 2 in, 1 out]
              n292 = Select(t="V17", s=w521, f="No Match" ("Message")) -> (s? t:f=w522:string)
            }
            frame "V17" {
              n293 = Wait (ms)(milliseconds to wait=w535) -> ()  [unwired: 1 out]
              n294 = local write "V 17"(FALSE ("V 3")) -> ()
              n295 = call "Control_Pump_Valves.vi"("Set state:"=FALSE, "Device"=Valve_Pump."V17") -> ("Good Reply"=w530:bool)  [unwired: 2 in, 1 out]
              n296 = Select(t="V19", s=w530, f="No Match" ("Message")) -> (s? t:f=w531:string)
            }
            frame "V19" {
              n297 = Wait (ms)(milliseconds to wait=w544) -> ()  [unwired: 1 out]
              n298 = local write "V 19"(FALSE ("V 3")) -> ()
              n299 = call "Control_Pump_Valves.vi"("Set state:"=FALSE, "Device"=Valve_Pump."V19") -> ("Good Reply"=w539:bool)  [unwired: 2 in, 1 out]
              n300 = Select(t="V30", s=w539, f="No Match" ("Message")) -> (s? t:f=w540:string)
            }
            frame "V30" {
              n301 = Wait (ms)(milliseconds to wait=w553) -> ()  [unwired: 1 out]
              n302 = local write "V 30"(TRUE ("V 3")) -> ()
              n303 = call "Control_Pump_Valves.vi"("Set state:"=TRUE, "Device"=Valve_Pump."V30") -> ("Good Reply"=w548:bool)  [unwired: 2 in, 1 out]
              n304 = Select(t="V32", s=w548, f="No Match" ("Message")) -> (s? t:f=w549:string)
            }
            frame "V32" {
              n305 = Wait (ms)(milliseconds to wait=w562) -> ()  [unwired: 1 out]
              n306 = local write "V 32"(TRUE ("V 3")) -> ()
              n307 = call "Control_Pump_Valves.vi"("Set state:"=TRUE, "Device"=Valve_Pump."V32") -> ("Good Reply"=w557:bool)  [unwired: 2 in, 1 out]
              n308 = Select(t="V33", s=w557, f="No Match" ("Message")) -> (s? t:f=w558:string)
            }
            frame "V33" {
              n309 = Wait (ms)(milliseconds to wait=w571) -> ()  [unwired: 1 out]
              n310 = local write "V 33"(FALSE ("V 3")) -> ()
              n311 = call "Control_Pump_Valves.vi"("Set state:"=FALSE, "Device"=Valve_Pump."V33") -> ("Good Reply"=w566:bool)  [unwired: 2 in, 1 out]
              n312 = Select(t="Pump A", s=w566, f="No Match" ("Message")) -> (s? t:f=w567:string)
            }
            frame "Pump A" {
              n313 = Wait (ms)(milliseconds to wait=w580) -> ()  [unwired: 1 out]
              n314 = local write "Pump A"(TRUE ("V 3")) -> ()
              n315 = call "Control_Pump_Valves.vi"("Set state:"=TRUE, "Device"=Valve_Pump."Pump A") -> ("Good Reply"=w575:bool)  [unwired: 2 in, 1 out]
              n316 = Select(t="Drain Tank", s=w575, f="No Match" ("Message")) -> (s? t:f=w576:string)
            }
          }
        }
      }
      frame "Drain Tank" {
        # "Drain Tank"
        n317 = for {
          N: 120 -> [_]
          tunnel: [w605] -> _ mode=indexing
          i -> [w605]
          # "Tank current level"
          # "Volumetric flow rate\n100 l/min"
          n318 = local read "Volume m^3*1000"() -> (w603:i32)
          n319 = Wait Until Next ms Multiple(millisecond multiple=u32 100) -> ()  [unwired: 1 out]
          n320 = Subtract(x=w603, y=100) -> (x-y=w604:i32)
          n321 = local write "Volume m^3*1000"(w604) -> ()
        }
        n322 = for {
          N: 121 -> [_]
          tunnel: [w595] -> w587
          # "Volume"
          # "Tank height"
          # "Area of tank"
          n323 = local read "Volume m^3*1000"() -> (w600:i32)
          n324 = Wait Until Next ms Multiple(millisecond multiple=u32 100 ("milliseconds to wait")) -> ()  [unwired: 1 out]
          n325 = Divide(x=w600, y=1000) -> (x/y=w598:dbl)
          n326 = Divide(x=w598, y=15) -> (x/y=w594:dbl)
          n327 = local write "Height of tank (m)"(w594) -> ()
          n328 = local write "Main tank"(w594) -> ()
          n329 = Equal?(x=w594, y=0.0) -> (x = y?=w595:bool)
        }
        n330 = case shown="True" w587 {
          tunnel: [FALSE ("OK") w592] -> w586
          frame False {
          }
          frame True {
            n331 = call "Display Message to User2"("Message"="Tank is empty. Close remaining Valves/Pumps?") -> ("OK"=w592:bool)  [unwired: 9 in, 1 out]
          }
        }
        n332 = Select(t="Close Remaining Ports", s=w586, f="No Match") -> (s? t:f=w583:string)
      }
      frame "Close Remaining Ports" {
        n333 = while {
          shift-left: "Pump A" ("Message") -> [w611]
          shift-right: [w612] -> w607
          stop <- w613 continue-if-true
          n334 = case shown="\"V32\"" w611 {
            tunnel: [FALSE TRUE TRUE FALSE] -> w613
            tunnel: ["Initialise" w624 w633 w643] -> w612
            tunnel: w611 -> [w616 _ _ _]
            tunnel: u32 250 ("milliseconds to wait") -> [_ w627 w636 w646]
            frame "No Match", Default {
              n335 = Current VI's Path() -> (path=w615:path)
              n336 = Format Into String(format string="The Case\"%s\" was not Matched\nin VI named\n'%s\"" ("Format String"), w616, w615) -> (resulting string=w619:string)  [unwired: 2 in, 1 out]
              n337 = One Button Dialog(message=w619, button name ("OK")="STOP") -> (true=w617:bool)
              n338 = Stop(stop? (T)=w617) -> ()
            }
            frame "Pump A" {
              n339 = Wait (ms)(milliseconds to wait=w627) -> ()  [unwired: 1 out]
              n340 = local write "Pump A"(FALSE ("Pump B")) -> ()
              n341 = call "Control_Pump_Valves.vi"("Set state:"=FALSE, "Device"=Valve_Pump."Pump A") -> ("Good Reply"=w623:bool)  [unwired: 2 in, 1 out]
              n342 = Select(t="V30", s=w623, f="No Match" ("Message")) -> (s? t:f=w624:string)
            }
            frame "V30" {
              n343 = Wait (ms)(milliseconds to wait=w636) -> ()  [unwired: 1 out]
              n344 = local write "V 30"(FALSE ("Pump B")) -> ()
              n345 = call "Control_Pump_Valves.vi"("Set state:"=FALSE, "Device"=Valve_Pump."V30") -> ("Good Reply"=w632:bool)  [unwired: 2 in, 1 out]
              n346 = Select(t="V32", s=w632, f="No Match" ("Message")) -> (s? t:f=w633:string)
            }
            frame "V32" {
              n347 = Wait (ms)(milliseconds to wait=w646) -> ()  [unwired: 1 out]
              n348 = local write "V 32"(FALSE ("Pump B")) -> ()
              n349 = local write "Drain Main Tank"(FALSE ("Drain Main Tank")) -> ()
              n350 = call "Control_Pump_Valves.vi"("Set state:"=FALSE, "Device"=Valve_Pump."V32") -> ("Good Reply"=w642:bool)  [unwired: 2 in, 1 out]
              n351 = Select(t="Start", s=w642, f="No Match" ("Message")) -> (s? t:f=w643:string)
            }
          }
        }
      }
    }
  }
  n352 = while {
    shift-left: "Start" -> [w651]
    shift-right: [w652] -> _
    stop <- w653 continue-if-true
    n353 = case shown="\"First Case\"" w651 {
      tunnel: [FALSE TRUE TRUE] -> w653
      tunnel: ["Initialise" w662 "Start"] -> w652
      tunnel: w651 -> [w656 _ _]
      tunnel: u32 250 ("milliseconds to wait") -> [_ _ w746]
      frame "No Match", Default {
        n354 = Current VI's Path() -> (path=w655:path)
        n355 = Format Into String(format string="The Case\"%s\" was not Matched\nin VI named\n'%s\"" ("Format String"), w656, w655) -> (resulting string=w659:string)  [unwired: 2 in, 1 out]
        n356 = One Button Dialog(message=w659, button name ("OK")="STOP") -> (true=w657:bool)
        n357 = Stop(stop? (T)=w657) -> ()
      }
      frame "Start" {
        n358 = Select(t="First Case", s="Manual Override", f="Start") -> (s? t:f=w662:string)
      }
      frame "First Case" {
        n359 = call "Control_Pump_Valves.vi"("Set state:"="V 3", "Device"=Valve_Pump."V3") -> ()  [unwired: 2 in, 2 out]
        n360 = call "Control_Pump_Valves.vi"("Set state:"="V 4", "Device"=Valve_Pump."V4") -> ()  [unwired: 2 in, 2 out]
        n361 = call "Control_Pump_Valves.vi"("Set state:"="V 2", "Device"=Valve_Pump."V2") -> ()  [unwired: 2 in, 2 out]
        n362 = call "Control_Pump_Valves.vi"("Set state:"="V 1", "Device"=Valve_Pump."V1") -> ()  [unwired: 2 in, 2 out]
        n363 = call "Control_Pump_Valves.vi"("Set state:"="V 5", "Device"=Valve_Pump."V5") -> ()  [unwired: 2 in, 2 out]
        n364 = call "Control_Pump_Valves.vi"("Set state:"="V 6", "Device"=Valve_Pump."V6") -> ()  [unwired: 2 in, 2 out]
        n365 = call "Control_Pump_Valves.vi"("Set state:"="V 8", "Device"=Valve_Pump."V8") -> ()  [unwired: 2 in, 2 out]
        n366 = call "Control_Pump_Valves.vi"("Set state:"="V 7", "Device"=Valve_Pump."V7") -> ()  [unwired: 2 in, 2 out]
        n367 = call "Control_Pump_Valves.vi"("Set state:"="V 9", "Device"=Valve_Pump."V9") -> ()  [unwired: 2 in, 2 out]
        n368 = call "Control_Pump_Valves.vi"("Set state:"="V 10", "Device"=Valve_Pump."V10") -> ()  [unwired: 2 in, 2 out]
        n369 = call "Control_Pump_Valves.vi"("Set state:"="V 11", "Device"=Valve_Pump."V11") -> ()  [unwired: 2 in, 2 out]
        n370 = call "Control_Pump_Valves.vi"("Set state:"="V 12", "Device"=Valve_Pump."V12") -> ()  [unwired: 2 in, 2 out]
        n371 = call "Control_Pump_Valves.vi"("Set state:"="V 16", "Device"=Valve_Pump."V16") -> ()  [unwired: 2 in, 2 out]
        n372 = call "Control_Pump_Valves.vi"("Set state:"="V 15", "Device"=Valve_Pump."V15") -> ()  [unwired: 2 in, 2 out]
        n373 = call "Control_Pump_Valves.vi"("Set state:"="V 14", "Device"=Valve_Pump."V14") -> ()  [unwired: 2 in, 2 out]
        n374 = call "Control_Pump_Valves.vi"("Set state:"="V 13", "Device"=Valve_Pump."V13") -> ()  [unwired: 2 in, 2 out]
        n375 = call "Control_Pump_Valves.vi"("Set state:"="V 20", "Device"=Valve_Pump."V20") -> ()  [unwired: 2 in, 2 out]
        n376 = call "Control_Pump_Valves.vi"("Set state:"="V 17", "Device"=Valve_Pump."V17") -> ()  [unwired: 2 in, 2 out]
        n377 = call "Control_Pump_Valves.vi"("Set state:"="V 18", "Device"=Valve_Pump."V18") -> ()  [unwired: 2 in, 2 out]
        n378 = call "Control_Pump_Valves.vi"("Set state:"="V 19", "Device"=Valve_Pump."V19") -> ()  [unwired: 2 in, 2 out]
        n379 = call "Control_Pump_Valves.vi"("Set state:"="V 21", "Device"=Valve_Pump."V21") -> ()  [unwired: 2 in, 2 out]
        n380 = call "Control_Pump_Valves.vi"("Set state:"="V 22", "Device"=Valve_Pump."V22") -> ()  [unwired: 2 in, 2 out]
        n381 = call "Control_Pump_Valves.vi"("Set state:"="V 23", "Device"=Valve_Pump."V23") -> ()  [unwired: 2 in, 2 out]
        n382 = call "Control_Pump_Valves.vi"("Set state:"="V 24", "Device"=Valve_Pump."V24") -> ()  [unwired: 2 in, 2 out]
        n383 = call "Control_Pump_Valves.vi"("Set state:"="V 25", "Device"=Valve_Pump."V25") -> ()  [unwired: 2 in, 2 out]
        n384 = call "Control_Pump_Valves.vi"("Set state:"="V 27", "Device"=Valve_Pump."V27") -> ()  [unwired: 2 in, 2 out]
        n385 = call "Control_Pump_Valves.vi"("Set state:"="V 26", "Device"=Valve_Pump."V26") -> ()  [unwired: 2 in, 2 out]
        n386 = call "Control_Pump_Valves.vi"("Set state:"="V 28", "Device"=Valve_Pump."V28") -> ()  [unwired: 2 in, 2 out]
        n387 = call "Control_Pump_Valves.vi"("Set state:"="V 29", "Device"=Valve_Pump."V29") -> ()  [unwired: 2 in, 2 out]
        n388 = call "Control_Pump_Valves.vi"("Set state:"="V 30", "Device"=Valve_Pump."V30") -> ()  [unwired: 2 in, 2 out]
        n389 = call "Control_Pump_Valves.vi"("Set state:"="V 31", "Device"=Valve_Pump."V31") -> ()  [unwired: 2 in, 2 out]
        n390 = call "Control_Pump_Valves.vi"("Set state:"="V 32", "Device"=Valve_Pump."V32") -> ()  [unwired: 2 in, 2 out]
        n391 = call "Control_Pump_Valves.vi"("Set state:"="V 33", "Device"=Valve_Pump."V33") -> ()  [unwired: 2 in, 2 out]
        n392 = call "Control_Pump_Valves.vi"("Set state:"="V 34", "Device"=Valve_Pump."V34") -> ()  [unwired: 2 in, 2 out]
        n393 = call "Control_Pump_Valves.vi"("Device"=Valve_Pump."V35") -> ()  [unwired: 3 in, 2 out]
        n394 = call "Control_Pump_Valves.vi"("Set state:"="V 36", "Device"=Valve_Pump."V36") -> ()  [unwired: 2 in, 2 out]
        n395 = call "Control_Pump_Valves.vi"("Set state:"="Pump C", "Device"=Valve_Pump."Pump C") -> ()  [unwired: 2 in, 2 out]
        n396 = call "Control_Pump_Valves.vi"("Set state:"="Pump A", "Device"=Valve_Pump."Pump A") -> ()  [unwired: 2 in, 2 out]
        n397 = call "Control_Pump_Valves.vi"("Set state:"="V 37", "Device"=Valve_Pump."V37") -> ()  [unwired: 2 in, 2 out]
        n398 = call "Control_Pump_Valves.vi"("Set state:"="Pump B", "Device"=Valve_Pump."Pump B") -> ()  [unwired: 2 in, 2 out]
        n399 = call "Control_Pump_Valves.vi"("Set state:"="Pump D", "Device"=Valve_Pump."Pump D") -> ()  [unwired: 2 in, 2 out]
        n400 = Wait (ms)(milliseconds to wait=w746) -> ()  [unwired: 1 out]
      }
    }
  }
